vi "load_parameters.vi"(4 "Create Data Folder (T)":bool=TRUE, 5 "Set Up Projector and Camera (T)":bool=TRUE, 6 "additional loaded parameters to write":string[][](array[string]), 8 "error in (no error)":errorcluster, 9 "StimulusObject Parameters":variant, 10 "StimulusObjectClassInput":refnum<class "StimulusObject.lvclass">, 11 "Tags":string) -> (0 "error out":errorcluster, 2 "Computer Found":bool, 3 "Parameters":T1 {"FW_WormLengthSD" format="%#.6f"})   [LabVIEW 2019]
uses:
  Parameters.ctl
  StimulusObject.lvclass
  <vilib>/AdvancedString/Delimited String to 1D String Array.vi
  ParametersGlobal.vi
  <vilib>/Utility/file.llb/Write Delimited Spreadsheet (string).vi
  <vilib>/vision/driver/NI_Vision_Acquisition_Software.lvlib
  <vilib>/vision/NI_Vision_Development_Module.lvlib
panel:
  out "Cores Utilized":u32
  out "Camera Frame Rate":dbl
  # "Faux Worm Drawing"
  # "Tracking"
  # "Temporal Calibration"
  # "Stimulus Generation"
  # "Median Filtering"
  # "Experimental Settings"
  # "Camera and Projector Settings"
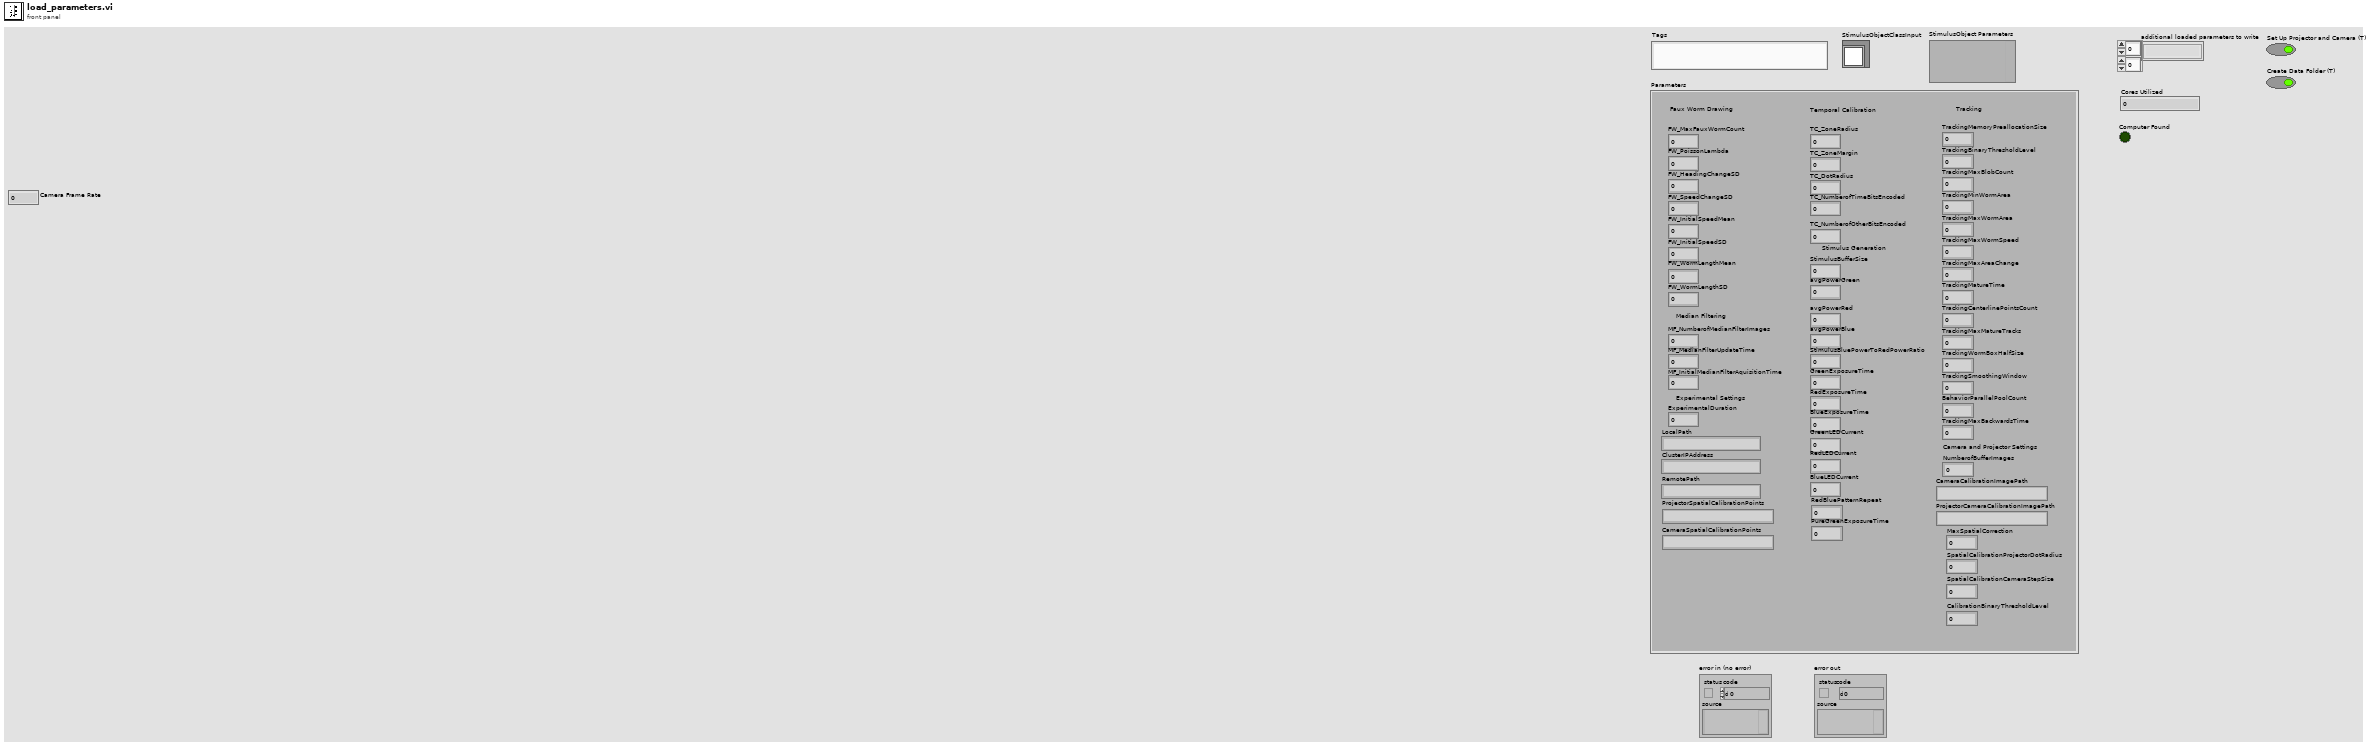
[diagram p1: front panel]
types:
  T1 = typedef "Parameters.ctl" = cluster{"FW_MaxFauxWormCount":i32, "FW_PoissonLambda":dbl, "FW_HeadingChangeSD":dbl, "FW_SpeedChangeSD":dbl, "FW_InitialSpeedMean":dbl, "FW_InitialSpeedSD":dbl, "FW_WormLengthMean":dbl, "FW_WormLengthSD":dbl, "MF_NumberofMedianFilterImages":i32, "MF_MedianFilterUpdateTime":i32, "MF_InitialMedianFilterAquisitionTime":dbl, "ExperimentalDuration":i32, "TC_ZoneRadius":i32, "TC_ZoneMargin":i32, "TC_DotRadius":dbl, "TC_NumberofTimeBitsEncoded":i32, "TC_NumberofOtherBitsEncoded":i32, "NumberofBufferImages":sgl, "CameraCalibrationImagePath":string, "ProjectorCameraCalibrationImagePath":string, "StimulusBufferSize":i32, "TrackingMemoryPreallocationSize":i32, "TrackingBinaryThresholdLevel":sgl, "TrackingMaxBlobCount":i32, "TrackingMinWormArea":dbl, "TrackingMaxWormArea":dbl, "TrackingMaxWormSpeed":dbl, "TrackingMaxAreaChange":dbl, "TrackingMatureTime":i32, "TrackingCenterlinePointsCount":i32, "TrackingMaxMatureTracks":i32, "TrackingWormBoxHalfSize":i32, "TrackingSmoothingWindow":i32, "BehaviorParallelPoolCount":i32, "LocalPath":string, "GreenExposureTime":i32, "RedExposureTime":i32, "BlueExposureTime":i32, "ClusterIPAddress":string, "RemotePath":string, "GreenLEDCurrent":u8, "RedLEDCurrent":u8, "BlueLEDCurrent":u8, "avgPowerGreen":sgl, "avgPowerRed":sgl, "avgPowerBlue":sgl, "StimulusBluePowerToRedPowerRatio":sgl, "TrackingMaxBackwardsTime":i32, "MaxSpatialCorrection":dbl, "ProjectorSpatialCalibrationPoints":string, "SpatialCalibrationProjectorDotRadius":i32, "SpatialCalibrationCameraStepSize":dbl, "CameraSpatialCalibrationPoints":string, "CalibrationBinaryThresholdLevel":dbl, "RedBluePatternRepeat":i32, "PureGreenExposureTime":i32}
  T2 = cluster{"Type":u32, "Version":u32, "Flags":u32, "SerialNumberHigh":u32, "SerialNumberLow":u32, "BusType":u32, "InterfaceName":string, "VendorName":string, "ModelName":string, "CameraFileName":string, "CameraAttributeURL":string}[]
  T3 = cluster{"Type":u32, "Version":u32, "Flags":u32, "SerialNumberHigh":u32, "SerialNumberLow":u32, "BusType":u32, "InterfaceName":string, "VendorName":string, "ModelName":string, "CameraFileName":string, "CameraAttributeURL":string}
  T4 = typedef "IMAQ Image.ctl" = refnum<image>
  T5 = typedef "Image Type" = u32
  T6 = enum16{"open", "replace", "create", "open or create", "replace or create", "replace or create with confirmation"}
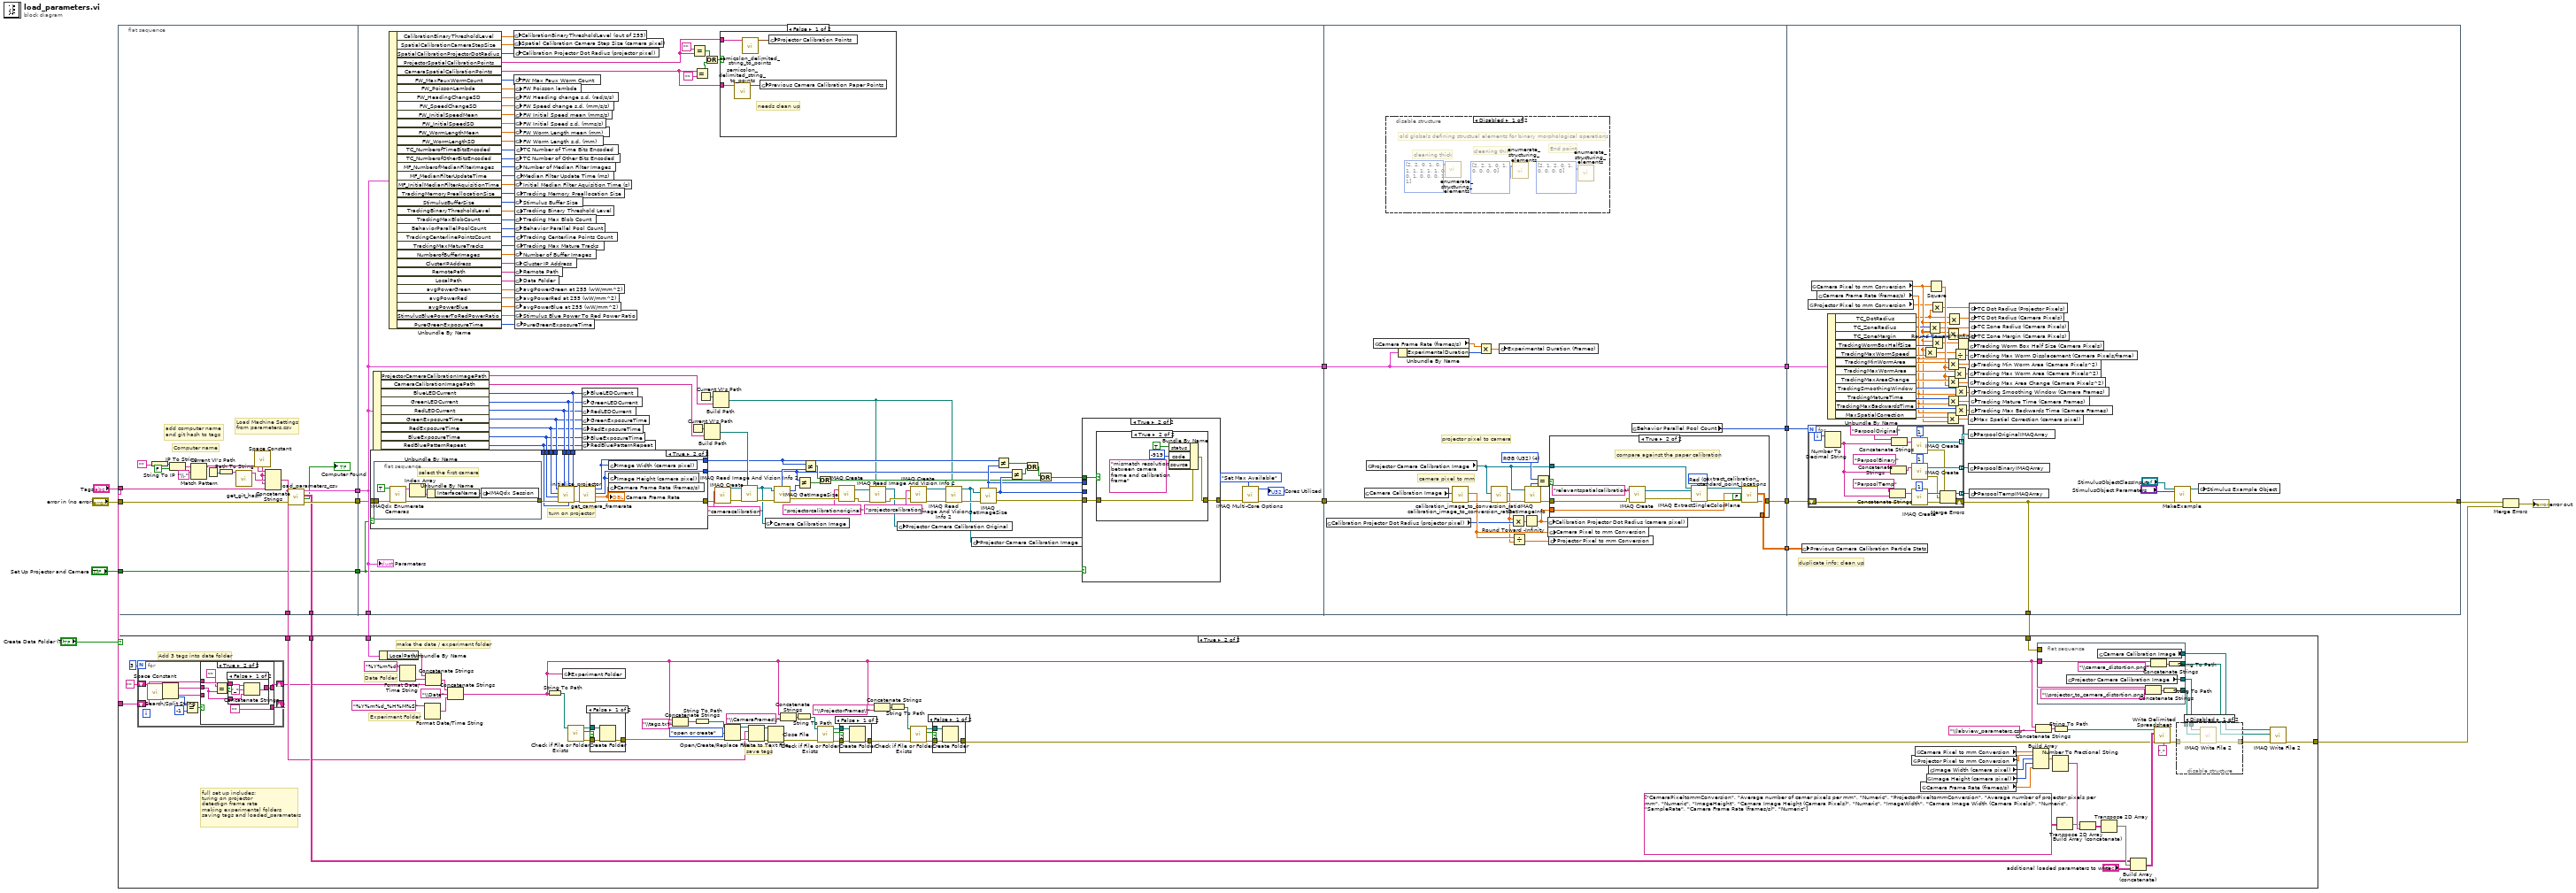
[diagram p0: block diagram]
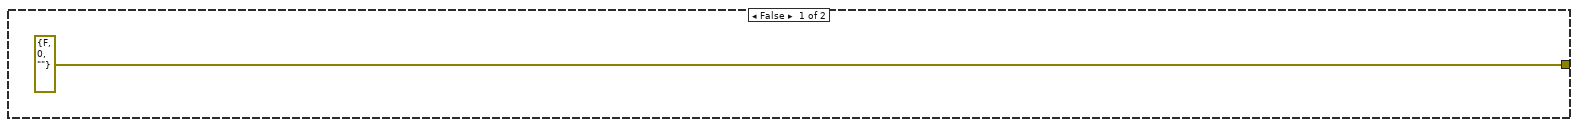
[diagram p2: hidden frame]
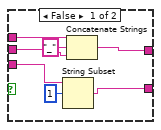
[diagram p7: hidden frame]
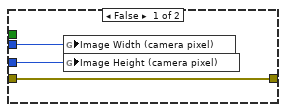
[diagram p10: hidden frame]
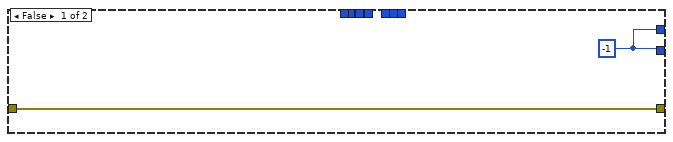
[diagram p12: hidden frame]
diagram:
  n1 = flat-sequence {
    tunnel: [w38] -> w19
    tunnel: "error in (no error)" -> [w23]
    tunnel: [w24] -> w18
    tunnel: "Tags" -> [w30]
    tunnel: [w26] -> w11
    tunnel: [w25] -> w10
    tunnel: [w22] -> w5
    tunnel: "Set Up Projector and Camera (T)" -> [w22]
    tunnel: w19 -> [w96]
    tunnel: [w87] -> w17
    tunnel: w18 -> [w97]
    tunnel: [w97] -> w14
    tunnel: [w97] -> w6
    tunnel: w5 -> [w73]
    tunnel: w17 -> [w187]
    tunnel: [w175] -> w16
    tunnel: [w183] -> w15
    tunnel: w14 -> [w183]
    tunnel: [w184] -> w13
    tunnel: [w172] -> w1
    tunnel: w16 -> [w226]
    tunnel: w15 -> [w247]
    tunnel: w13 -> [w225]
    tunnel: [w214] -> w9
    tunnel: [w218] -> w2
    tunnel: w1 -> [w217]
    frame #0 {
      # "add computer name \nand git hash to tags"
      # "Computer name"
      # "Load Machine Settings\nfrom parameters.csv"
      n2 = String To IP(1:"") -> (0:w37:u32)
      n3 = IP To String(1:FALSE, 2:w37) -> (0:w34:string)
      n4 = Match Pattern(string=w34, regular expression="\\.") -> (before substring=w28:string)  [unwired: 1 in, 3 out]
      n5 = Current VI's Path() -> (path=w32:path)
      n6 = Path To String(path=w32) -> (string=w31:string)
      n7 = call "get_git_hash.vi"("VI folder"=w31) -> ("github hash"=w29:string)  [unwired: 10 in]
      n8 = call <vilib>:"Space Constant.vi"() -> ("String"=w27:string)
      n9 = Concatenate Strings(w28, w27, w29, w27, w30) -> (w25:string)
      n10 = call "load_parameters_csv.vi"("error in (no error)"=w23, "Tags In"=w25) -> ("error out"=w38:errorcluster, "Computer Found"=→"Computer Found":bool, "Loaded Params"=w26:string[][], "Parameters Out"=w24:T1)  [unwired: 6 in]
    }
    frame #1 {
      n11 = Unbundle By Name(w97) -> ("ProjectorCameraCalibrationImagePath"=w67:string, "CameraCalibrationImagePath"=w119:string, "BlueLEDCurrent"=w46:u8, "GreenLEDCurrent"=w45:u8, "RedLEDCurrent"=w44:u8, "GreenExposureTime"=w43:i32, "RedExposureTime"=w42:i32, "BlueExposureTime"=w41:i32, "RedBluePatternRepeat"=w40:i32)
      n12 = case shown="True" w73 {
        tunnel: w96 -> [w146 w151]
        tunnel: [w146 w158] -> w95
        tunnel: w43 -> [_ w157]
        tunnel: w42 -> [_ w156]
        tunnel: w41 -> [_ w155]
        tunnel: w44 -> [_ w154]
        tunnel: w46 -> [_ w153]
        tunnel: w45 -> [_ w152]
        tunnel: [w145 w149] -> w66
        tunnel: [w145 w148] -> w65
        tunnel: w40 -> [_ w147]
        frame False {
          w145 = -1 ("Image Width (camera pixel)")
        }
        frame True {
          # "turn on projector"
          n13 = flat-sequence {
            tunnel: w151 -> [w163]
            tunnel: [w162] -> w150
            frame #0 {
              # "select the first camera"
              n14 = call <vilib>:"IMAQdx Enumerate Cameras.vi"("error in"=w163, "Connected Only? (Yes)"=TRUE) -> ("error out"=w162:errorcluster, "Camera Information Array"=w166:T2)  [unwired: 8 in]
              n15 = Index Array(array=w166) -> (element=w165:T3)  [unwired: 1 in]
              n16 = Unbundle By Name(w165) -> ("InterfaceName"=w161:string)
              n17 = global write "ParametersGlobal.vi" "IMAQdx Session"(w161) -> ()
            }
          }
          n18 = call "initialize_projector.vi"("BlueCurrent"=w153, "RedBluePatternRepeat"=w147, "GreenCurrent"=w152, "RedCurrent"=w154, "error in"=w150, "blue exp_time_us"=w155, "red exp_time_us"=w156, "green exp_time_us"=w157) -> ("error out"=w159:errorcluster)  [unwired: 3 in]
          n19 = call "get_camera_framerate.vi"("error in"=w159) -> ("error out"=w158:errorcluster, "Camera Frame Rate"=w160:dbl, "Y Resolution"=w148:i32, "X Resolution"=w149:i32)  [unwired: 7 in]
          "Camera Frame Rate" <- w160
          n20 = global write "ParametersGlobal.vi" "Image Width (camera pixel)"(w149) -> ()
          n21 = global write "ParametersGlobal.vi" "Image Height (camera pixel)"(w148) -> ()
          n22 = global write "ParametersGlobal.vi" "Camera Frame Rate (frames/s)"(w160) -> ()
        }
      }
      n23 = Unbundle By Name(w97) -> ("CalibrationBinaryThresholdLevel"=w47:dbl, "SpatialCalibrationCameraStepSize"=w61:dbl, "SpatialCalibrationProjectorDotRadius"=w62:i32, "ProjectorSpatialCalibrationPoints"=w63:string, "CameraSpatialCalibrationPoints"=w48:string, "FW_MaxFauxWormCount"=w109:i32, "FW_PoissonLambda"=w110:dbl, "FW_HeadingChangeSD"=w111:dbl, "FW_SpeedChangeSD"=w112:dbl, "FW_InitialSpeedMean"=w113:dbl, "FW_InitialSpeedSD"=w114:dbl, "FW_WormLengthMean"=w115:dbl, "FW_WormLengthSD"=w116:dbl, "TC_NumberofTimeBitsEncoded"=w117:i32, "TC_NumberofOtherBitsEncoded"=w118:i32, "MF_NumberofMedianFilterImages"=w108:i32, "MF_MedianFilterUpdateTime"=w107:i32, "MF_InitialMedianFilterAquisitionTime"=w106:dbl, "TrackingMemoryPreallocationSize"=w105:i32, "StimulusBufferSize"=w104:i32, "TrackingBinaryThresholdLevel"=w103:sgl, "TrackingMaxBlobCount"=w102:i32, "BehaviorParallelPoolCount"=w101:i32, "TrackingCenterlinePointsCount"=w100:i32, "TrackingMaxMatureTracks"=w99:i32, "NumberofBufferImages"=w98:sgl, "ClusterIPAddress"=w94:string, "RemotePath"=w93:string, "LocalPath"=w92:string, "avgPowerGreen"=w88:sgl, "avgPowerRed"=w89:sgl, "avgPowerBlue"=w90:sgl, "StimulusBluePowerToRedPowerRatio"=w91:sgl, "PureGreenExposureTime"=w39:i32)
      n24 = global write "ParametersGlobal.vi" "CalibrationBinaryThresholdLevel (out of 255)"(w47) -> ()
      n25 = global write "ParametersGlobal.vi" "Spatial Calibration Camera Step Size (camera pixel)"(w61) -> ()
      n26 = global write "ParametersGlobal.vi" "Calibration Projector Dot Radius (projector pixel)"(w62) -> ()
      n27 = global write "ParametersGlobal.vi" "FW Max Faux Worm Count"(w109) -> ()
      n28 = global write "ParametersGlobal.vi" "FW Poisson lambda"(w110) -> ()
      n29 = global write "ParametersGlobal.vi" "FW Heading change s.d. (rad/s/s)"(w111) -> ()
      n30 = global write "ParametersGlobal.vi" "FW Speed change s.d. (mm/s/s)"(w112) -> ()
      n31 = global write "ParametersGlobal.vi" "FW Initial Speed mean (mms/s)"(w113) -> ()
      n32 = global write "ParametersGlobal.vi" "FW Initial Speed s.d. (mms/s)"(w114) -> ()
      n33 = global write "ParametersGlobal.vi" "FW Worm Length mean (mm)"(w115) -> ()
      n34 = global write "ParametersGlobal.vi" "FW Worm Length s.d. (mm)"(w116) -> ()
      n35 = global write "ParametersGlobal.vi" "TC Number of Other Bits Encoded"(w118) -> ()
      n36 = global write "ParametersGlobal.vi" "Number of Median Filter Images"(w108) -> ()
      n37 = global write "ParametersGlobal.vi" "Initial Median Filter Aquisition Time (s)"(w106) -> ()
      n38 = global write "ParametersGlobal.vi" "Stimulus Buffer Size"(w104) -> ()
      n39 = global write "ParametersGlobal.vi" "Tracking Max Blob Count"(w102) -> ()
      n40 = global write "ParametersGlobal.vi" "Behavior Parallel Pool Count"(w101) -> ()
      n41 = global write "ParametersGlobal.vi" "Number of Buffer Images"(w98) -> ()
      n42 = global write "ParametersGlobal.vi" "Cluster IP Address"(w94) -> ()
      n43 = global write "ParametersGlobal.vi" "Remote Path"(w93) -> ()
      n44 = global write "ParametersGlobal.vi" "Data Folder"(w92) -> ()
      n45 = global write "ParametersGlobal.vi" "avgPowerGreen at 255 (wW/mm^2)"(w88) -> ()
      n46 = global write "ParametersGlobal.vi" "avgPowerRed at 255 (wW/mm^2)"(w89) -> ()
      n47 = global write "ParametersGlobal.vi" "avgPowerBlue at 255 (wW/mm^2)"(w90) -> ()
      n48 = global write "ParametersGlobal.vi" "Stimulus Blue Power To Red Power Ratio"(w91) -> ()
      n49 = global write "ParametersGlobal.vi" "TC Number of Time Bits Encoded"(w117) -> ()
      n50 = global write "ParametersGlobal.vi" "Median Filter Update Time (ms)"(w107) -> ()
      n51 = global write "ParametersGlobal.vi" "Tracking Memory Preallocation Size"(w105) -> ()
      n52 = global write "ParametersGlobal.vi" "Tracking Binary Threshold Level"(w103) -> ()
      n53 = global write "ParametersGlobal.vi" "Tracking Centerline Points Count"(w100) -> ()
      n54 = global write "ParametersGlobal.vi" "Tracking Max Mature Tracks"(w99) -> ()
      n55 = global write "ParametersGlobal.vi" "PureGreenExposureTime"(w39) -> ()
      n56 = global write "ParametersGlobal.vi" "BlueLEDCurrent"(w46) -> ()
      n57 = global write "ParametersGlobal.vi" "GreenLEDCurrent"(w45) -> ()
      n58 = global write "ParametersGlobal.vi" "RedLEDCurrent"(w44) -> ()
      n59 = global write "ParametersGlobal.vi" "GreenExposureTime"(w43) -> ()
      n60 = global write "ParametersGlobal.vi" "RedExposureTime"(w42) -> ()
      n61 = global write "ParametersGlobal.vi" "BlueExposureTime"(w41) -> ()
      n62 = global write "ParametersGlobal.vi" "RedBluePatternRepeat"(w40) -> ()
      n63 = Current VI's Path() -> (path=w124:path)
      n64 = Equal?(x="", y=w63) -> (x = y?=w51:bool)
      n65 = Equal?(x=w48, y="") -> (x = y?=w50:bool)
      n66 = Current VI's Path() -> (path=w128:path)
      n67 = Or(x=w51, y=w50) -> (x .or. y?=w49:bool)
      n68 = Build Path(base path=w124, name or relative path=w119) -> (appended path=w121:path)
      n69 = Build Path(base path=w128, name or relative path=w67) -> (appended path=w54:path)
      n70 = call "IMAQ Create"("Image Name"="cameracalibration", "error in (no error)"=w95) -> ("New Image"=w123:T4, "error out"=w122:errorcluster)  [unwired: 3 in]
      n71 = case shown="False" w49 {
        tunnel: w63 -> [w132 _]
        tunnel: w48 -> [w130 _]
        frame False {
          # "needs clean up"
          n72 = call "semicolon_delimited_string_to_points.vi"("delimited string"=w130) -> ("Array"=w129:cluster{"X":dbl, "Y":dbl}[])  [unwired: 10 in]
          n73 = call "semicolon_delimited_string_to_points.vi"("delimited string"=w132) -> ("Array"=w131:cluster{"X":dbl, "Y":dbl}[])  [unwired: 10 in]
          n74 = global write "ParametersGlobal.vi" "Previous Camera Calibration Paper Points"(w129) -> ()
          n75 = global write "ParametersGlobal.vi" "Projector Calibration Points"(w131) -> ()
        }
        frame True {
        }
      }
      n76 = call "IMAQ Read Image And Vision Info 2"("File Path"=w121, "error in (no error)"=w122, "Image"=w123) -> ("error out"=w84:errorcluster, "Image Out"=w81:T4)  [unwired: 6 in, 1 out]
      n77 = global write "ParametersGlobal.vi" "Camera Calibration Image"(w81) -> ()
      n78 = call "IMAQ GetImageSize"("Image"=w81, "error in (no error)"=w84) -> ("Y Resolution"=w82:i32, "X Resolution"=w83:i32, "error out"=w59:errorcluster)  [unwired: 2 in]
      n79 = Not Equal?(x=w65, y=w82) -> (x != y?=w78:bool)
      n80 = Not Equal?(x=w66, y=w83) -> (x != y?=w77:bool)
      n81 = Or(x=w77, y=w78) -> (x .or. y?=w60:bool)
      n82 = call "IMAQ Create"("Image Name"="projectorcalibrationoriginal", "error in (no error)"=w59) -> ("New Image"=w56:T4, "error out"=w57:errorcluster)  [unwired: 3 in]
      n83 = call "IMAQ Read Image And Vision Info 2"("File Path"=w54, "error in (no error)"=w57, "Image"=w56) -> ("error out"=w55:errorcluster, "Image Out"=w53:T4)  [unwired: 6 in, 1 out]
      n84 = global write "ParametersGlobal.vi" "Projector Camera Calibration Original"(w53) -> ()
      n85 = call "IMAQ Create"("Image Name"="projectorcalibration", "error in (no error)"=w55) -> ("New Image"=w126:T4, "error out"=w125:errorcluster)  [unwired: 3 in]
      n86 = call "IMAQ Read Image And Vision Info 2"("File Path"=w54, "error in (no error)"=w125, "Image"=w126) -> ("error out"=w80:errorcluster, "Image Out"=w79:T4)  [unwired: 6 in, 1 out]
      n87 = global write "ParametersGlobal.vi" "Projector Camera Calibration Image"(w79) -> ()
      n88 = call "IMAQ GetImageSize"("Image"=w79, "error in (no error)"=w80) -> ("Y Resolution"=w70:i32, "X Resolution"=w69:i32, "error out"=w72:errorcluster)  [unwired: 2 in]
      n89 = Not Equal?(x=w66, y=w69) -> (x != y?=w76:bool)
      n90 = Not Equal?(x=w65, y=w70) -> (x != y?=w75:bool)
      n91 = Or(x=w76, y=w75) -> (x .or. y?=w74:bool)
      n92 = Or(x=w74, y=w60) -> (x .or. y?=w68:bool)
      n93 = case shown="True" w73 {
        tunnel: w72 -> [w135 w137]
        tunnel: [w135 w136] -> w71
        tunnel: w70 -> [w134 _]
        tunnel: w69 -> [w133 _]
        tunnel: w68 -> [_ w138]
        frame False {
          n94 = global write "ParametersGlobal.vi" "Image Width (camera pixel)"(w133) -> ()
          n95 = global write "ParametersGlobal.vi" "Image Height (camera pixel)"(w134) -> ()
        }
        frame True {
          n96 = case shown="True" w138 {
            tunnel: w137 -> [w139 w141]
            tunnel: [w139 w140] -> w136
            frame False {
              # "all resolutions match"
            }
            frame True {
              n97 = Bundle By Name(cluster=w141, "status"=TRUE, "code"=-919, "source"="mismatch resolution between camera frame and calibration frame") -> (w140:errorcluster)
            }
          }
        }
      }
      n98 = call "IMAQ Multi-Core Options"("Get/Set Number of Cores (Get)"=enum32{"Get", "Set", "Set Max Available"}."Set Max Available", "error in (no error)"=w71) -> ("error out"=w87:errorcluster, "Cores Utilized"=→"Cores Utilized":u32)  [unwired: 8 in]
      "Parameters" <- w97
    }
    frame #2 {
      w176 = T5 4 items=["Grayscale (U8)", "Grayscale (I16)", "Grayscale (SGL)", "Complex (CSG)", "RGB (U32)", "HSL (U32)", "RGB (U64)", "Grayscale (U16)"] ("Image Type")
      # "projector pixel to camera"
      # "camera pixel to mm"
      n99 = global read "ParametersGlobal.vi" "Calibration Projector Dot Radius (projector pixel)"() -> (w170:i32)
      n100 = global read "ParametersGlobal.vi" "Camera Calibration Image"() -> (w186:T4)
      n101 = global read "ParametersGlobal.vi" "Projector Camera Calibration Image"() -> (w171:T4)
      n102 = global read "ParametersGlobal.vi" "Camera Frame Rate (frames/s)"() -> (w182:sgl)
      n103 = disable-structure shown="Disabled" {
        frame Disabled {
          # "old globals defining structual elements for binary morphological operations"
          # "End point"
          # "cleaning thin"
          # "cleaning thick"
          n104 = call "enumerate_structuring_elements.vi"("Structuring Elements"=i32[][][] [[[2, 2, 0], [1, 0, 1], [1, 1, 1]], [[1, 0, 0], [1, 0, 0], [0, 1, 1]]]) -> ()  [unwired: 4 in, 1 out]
          n105 = call "enumerate_structuring_elements.vi"("Structuring Elements"=i32[][][] [[[2, 2, 1], [0, 1, 0], [0, 0, 0]]]) -> ()  [unwired: 4 in, 1 out]
          n106 = call "enumerate_structuring_elements.vi"("Structuring Elements"=i32[][][] [[[2, 1, 2], [0, 1, 0], [0, 0, 0]]]) -> ()  [unwired: 4 in, 1 out]
        }
        frame Enabled {
        }
      }
      n107 = Unbundle By Name(w183) -> ("ExperimentalDuration"=w181:i32)
      n108 = call "calibration_image_to_conversion_ratio.vi"("error in (no error)"=w187, "Calibration Image"=w186) -> ("error out"=w188:errorcluster, "conversion ratio"=w179:dbl)  [unwired: 8 in]
      n109 = Multiply(x=w182, y=w181) -> (x*y=w180:sgl)
      n110 = call "calibration_image_to_conversion_ratio.vi"("error in (no error)"=w188, "Calibration Image"=w171) -> ("error out"=w178:errorcluster, "conversion ratio"=w169:dbl)  [unwired: 8 in]
      n111 = global write "ParametersGlobal.vi" "Experimental Duration (Frames)"(w180) -> ()
      n112 = Multiply(x=w169, y=w170) -> (x*y=w168:dbl)
      n113 = Divide(x=w179, y=w169) -> (x/y=w185:dbl)
      n114 = Round Toward -Infinity(1:w168) -> (0:w167:dbl)
      n115 = call "IMAQ GetImageInfo"("error in (no error)"=w178, "Image"=w171) -> ("error out"=w174:errorcluster, "Image Type"=w177:T5)  [unwired: 2 in, 6 out]
      n116 = Equal?(x=w176, y=w177) -> (x = y?=w173:bool)
      n117 = global write "ParametersGlobal.vi" "Calibration Projector Dot Radius (camera pixel)"(w167) -> ()
      n118 = global write "ParametersGlobal.vi" "Camera Pixel to mm Conversion"(w179) -> ()
      n119 = global write "ParametersGlobal.vi" "Projector Pixel to mm Conversion"(w185) -> ()
      n120 = case shown="True" w173 {
        tunnel: [w189 w195] -> w175
        tunnel: w174 -> [w189 w199]
        tunnel: w171 -> [_ w196]
        tunnel: [_ w197] -> w172
        tunnel: w167 -> [_ w194]
        frame False {
        }
        frame True {
          w191 = 0 items=["Red", "Green", "Blue", "Hue", "Saturation", "Luminance", "Value", "Intensity"] ("Color Plane")
          # "compare against the paper calibration"
          n121 = call "IMAQ Create"("Image Name"="relevantspatialcalibration", "error in (no error)"=w199) -> ("New Image"=w192:T4, "error out"=w193:errorcluster)  [unwired: 3 in]
          n122 = call "IMAQ ExtractSingleColorPlane"("Color Plane"=w191, "error in (no error)"=w193, "Image Dst"=w192, "Image Src"=w196) -> ("error out"=w200:errorcluster, "Image Dst Out"=w201:T4)  [unwired: 6 in]
          n123 = call "extract_calibration_standard_point_locations.vi"("error in (no error)"=w200, "Agar (T) Paper (F)"=FALSE, "expected dot radius (camera pixels)"=w194, "Image Src"=w201) -> ("error out"=w195:errorcluster, "Particle Measurements (Pixels)"=w197:dbl[][])  [unwired: 5 in, 1 out]
        }
      }
      n124 = global read "ParametersGlobal.vi" "Behavior Parallel Pool Count"() -> (w184:i32)
    }
    frame #3 {
      # "duplicate info: clean up"
      n125 = global write "ParametersGlobal.vi" "Previous Camera Calibration Particle Stats"(w217) -> ()
      n126 = global read "ParametersGlobal.vi" "Projector Pixel to mm Conversion"() -> (w206:sgl)
      n127 = for {
        N: w225 -> [_]
        shift-right: [w260] -> w218
        shift-left: w226 -> [w251]
        tunnel: [w264] -> w227 mode=indexing
        tunnel: [w259] -> w228 mode=indexing
        tunnel: [w256] -> w229 mode=indexing
        i -> [w261]
        n128 = Number To Decimal String(number=w261) -> (decimal integer string=w255:string)  [unwired: 1 in]
        n129 = Concatenate Strings("ParpoolTemp", w255) -> (w258:string)
        n130 = Concatenate Strings("ParpoolBinary", w255) -> (w262:string)
        n131 = Concatenate Strings("ParpoolOriginal", w255) -> (w265:string)
        n132 = call "IMAQ Create"("Border Size"=1, "Image Name"=w262) -> ("New Image"=w259:T4, "error out"=w253:errorcluster)  [unwired: 3 in]
        n133 = call "IMAQ Create"("Border Size"=1, "Image Name"=w258, "error in (no error)"=w251) -> ("New Image"=w256:T4, "error out"=w254:errorcluster)  [unwired: 2 in]
        n134 = call "IMAQ Create"("Border Size"=1, "Image Name"=w265) -> ("New Image"=w264:T4, "error out"=w252:errorcluster)  [unwired: 3 in]
        n135 = Merge Errors(w252, w253, w254) -> (w260:errorcluster)
      }
      n136 = global read "ParametersGlobal.vi" "Camera Pixel to mm Conversion"() -> (w211:sgl)
      n137 = global read "ParametersGlobal.vi" "Camera Frame Rate (frames/s)"() -> (w221:sgl)
      n138 = Unbundle By Name(w247) -> ("TC_DotRadius"=w207:dbl, "TC_ZoneRadius"=w213:i32, "TC_ZoneMargin"=w212:i32, "TrackingWormBoxHalfSize"=w236:i32, "TrackingMaxWormSpeed"=w239:dbl, "TrackingMinWormArea"=w246:dbl, "TrackingMaxWormArea"=w245:dbl, "TrackingMaxAreaChange"=w242:dbl, "TrackingSmoothingWindow"=w233:i32, "TrackingMatureTime"=w231:i32, "TrackingMaxBackwardsTime"=w222:i32, "MaxSpatialCorrection"=w216:dbl)
      n139 = Multiply(x=w211, y=w239) -> (x*y=w238:dbl)
      n140 = Multiply(x=w213, y=w211) -> (x*y=w209:sgl)
      n141 = Square(x=w211) -> (x^2=w241:sgl)
      n142 = Multiply(x=w206, y=w207) -> (x*y=w205:dbl)
      n143 = Multiply(x=w211, y=w236) -> (x*y=w235:sgl)
      n144 = Multiply(x=w216, y=w211) -> (x*y=w215:dbl)
      n145 = Multiply(x=w211, y=w212) -> (x*y=w208:sgl)
      n146 = Multiply(x=w246, y=w241) -> (x*y=w244:dbl)
      n147 = Multiply(x=w242, y=w241) -> (x*y=w240:dbl)
      n148 = Multiply(x=w231, y=w221) -> (x*y=w230:sgl)
      n149 = Multiply(x=w207, y=w211) -> (x*y=w210:dbl)
      n150 = Multiply(x=w245, y=w241) -> (x*y=w243:dbl)
      n151 = Divide(x=w238, y=w221) -> (x/y=w237:dbl)
      n152 = Multiply(x=w233, y=w221) -> (x*y=w232:sgl)
      n153 = Multiply(x=w222, y=w221) -> (x*y=w220:sgl)
      n154 = Round Toward +Infinity(x=w235) -> (ceil(x): smallest int >= x=w234:sgl)
      n155 = global write "ParametersGlobal.vi" "Tracking Worm Box Half Size (Camera Pixels)"(w234) -> ()
      n156 = global write "ParametersGlobal.vi" "Tracking Max Worm Displacement (Camera Pixels/frame)"(w237) -> ()
      n157 = global write "ParametersGlobal.vi" "Tracking Max Worm Area (Camera Pixels^2)"(w243) -> ()
      n158 = global write "ParametersGlobal.vi" "Tracking Max Area Change (Camera Pixels^2)"(w240) -> ()
      n159 = global write "ParametersGlobal.vi" "Max Spatial Correction (camera pixel)"(w215) -> ()
      n160 = global write "ParametersGlobal.vi" "ParpoolOriginalIMAQArray"(w227) -> ()
      n161 = global write "ParametersGlobal.vi" "ParpoolBinaryIMAQArray"(w228) -> ()
      n162 = global write "ParametersGlobal.vi" "TC Dot Radius (Projector Pixels)"(w205) -> ()
      n163 = global write "ParametersGlobal.vi" "TC Dot Radius (Camera Pixels)"(w210) -> ()
      n164 = global write "ParametersGlobal.vi" "TC Zone Radius (Camera Pixels)"(w209) -> ()
      n165 = global write "ParametersGlobal.vi" "TC Zone Margin (Camera Pixels)"(w208) -> ()
      n166 = global write "ParametersGlobal.vi" "Tracking Min Worm Area (Camera Pixels^2)"(w244) -> ()
      n167 = global write "ParametersGlobal.vi" "Tracking Smoothing Window (Camera Frames)"(w232) -> ()
      n168 = global write "ParametersGlobal.vi" "ParpoolTempIMAQArray"(w229) -> ()
      n169 = global write "ParametersGlobal.vi" "Tracking Mature Time (Camera Frames)"(w230) -> ()
      n170 = global write "ParametersGlobal.vi" "Tracking Max Backwards Time (Camera Frames)"(w220) -> ()
      n171 = call-dynamic "MakeExample.vi"("error in (no error)"=w218, "StimulusObject Parameters"="StimulusObject Parameters", "StimulusObject in"="StimulusObjectClassInput") -> ("error out"=w214:errorcluster, "StimulusObject out"=w223:refnum<class "StimulusObject.lvclass">)  [unwired: 7 in]
      n172 = global write "ParametersGlobal.vi" "Stimulus Example Object"(w223) -> ()
    }
  }
  n173 = case shown="True" "Create Data Folder (T)" {
    tunnel: "Tags" -> [_ w335]
    tunnel: w11 -> [_ w284]
    tunnel: w10 -> [_ w282]
    tunnel: [errorcluster {"status"=FALSE, "code"=0, "source"=""} ("error out") w275] -> w7
    tunnel: w6 -> [_ w279]
    tunnel: w2 -> [_ w268]
    frame False {
    }
    frame True {
      # "full set up includes:\nturing on projector\ndetectign frame rate\nmaking experimental folders\nsaving tags and loaded_parameters"
      # "save tags"
      # "make the date / experiment folder"
      # "Experiment Folder"
      # "Date Folder"
      # "Add 3 tags into date folder"
      n174 = for {
        N: 3 -> [_]
        shift-right: [w362] -> _
        shift-left: w335 -> [w371]
        shift-right: [w364] -> w278
        shift-left: "" -> [w369]
        n175 = call <vilib>:"Space Constant.vi"() -> ("String"=w370:string)
        n176 = Search/Split String(string=w371, search string/char (-)=w370) -> (substring before match=w368:string, match + rest of string=w367:string, offset of match=w366:i32)  [unwired: 1 in]
        n177 = Equal?(x=w366, y=-1) -> (x = y?=w363:bool)
        n178 = case shown="True" w363 {
          tunnel: w369 -> [w372 w382]
          tunnel: w368 -> [w373 w379]
          tunnel: w367 -> [w374 _]
          tunnel: [w376 ""] -> w362
          tunnel: [w375 w381] -> w364
          frame False {
            n179 = String Subset(string=w374, offset (0)=1) -> (substring=w376:string)  [unwired: 1 in]
            n180 = Concatenate Strings(w372, "_", w373) -> (w375:string)
          }
          frame True {
            n181 = Equal?(x="", y=w379) -> (x = y?=w383:bool)
            n182 = case shown="False" w383 {
              tunnel: w382 -> [w386 w389]
              tunnel: [w387 w389] -> w381
              tunnel: w379 -> [w385 _]
              frame False {
                n183 = Concatenate Strings(w386, "_", w385) -> (w387:string)
              }
              frame True {
              }
            }
          }
        }
      }
      n184 = Unbundle By Name(w279) -> ("LocalPath"=w269:string)
      n185 = Format Date/Time String(time format string (%c)="%Y%m%d") -> (date/time string=w330:string)  [unwired: 2 in]
      n186 = Format Date/Time String(time format string (%c)="%Y%m%d_%H%M%S") -> (date/time string=w329:string)  [unwired: 2 in]
      n187 = Concatenate Strings(w269, w330, w278) -> (w331:string)
      n188 = Concatenate Strings(w331, "\\Data", w329) -> (w270:string)
      n189 = String To Path(string=w270) -> (path=w328:path)
      n190 = global write "ParametersGlobal.vi" "Experiment Folder"(w270) -> ()
      n191 = call <vilib>:"Check if File or Folder Exists.vi"("path"=w328) -> ("error out"=w332:errorcluster, "file or folder exists?"=w326:bool, "dup path"=w327:path)  [unwired: 8 in]
      n192 = case shown="False" w326 {
        tunnel: w327 -> [w360 _]
        tunnel: [w359 w361] -> w308
        tunnel: w332 -> [w358 w361]
        frame False {
          n193 = Create Folder(path (use dialog)=w360, error in=w358) -> (error out=w359:errorcluster)  [unwired: 1 in, 2 out]
        }
        frame True {
        }
      }
      n194 = Concatenate Strings(w270, "\\tags.txt" ("string")) -> (w312:string)
      n195 = String To Path(string=w312) -> (path=w315:path)
      n196 = Open/Create/Replace File(file path (use dialog)=w315, error in=w308, operation (0:open)=T6."open or create") -> (refnum out=w314:refnum<file>, error out=w313:errorcluster)  [unwired: 3 in, 1 out]
      n197 = Write to Text File(file (use dialog)=w314, text=w282, error in=w313) -> (refnum out=w316:refnum<file>, error out=w317:errorcluster)  [unwired: 1 in, 1 out]
      n198 = Close File(refnum=w316, error in=w317) -> (error out=w320:errorcluster)  [unwired: 1 out]
      n199 = Concatenate Strings(w270, "\\CameraFrames\\" ("string")) -> (w321:string)
      n200 = String To Path(string=w321) -> (path=w322:path)
      n201 = call <vilib>:"Check if File or Folder Exists.vi"("error in (no error)"=w320, "path"=w322) -> ("error out"=w323:errorcluster, "file or folder exists?"=w319:bool, "dup path"=w318:path)  [unwired: 7 in]
      n202 = case shown="False" w319 {
        tunnel: w318 -> [w356 _]
        tunnel: [w355 w357] -> w283
        tunnel: w323 -> [w354 w357]
        frame False {
          n203 = Create Folder(path (use dialog)=w356, error in=w354) -> (error out=w355:errorcluster)  [unwired: 1 in, 2 out]
        }
        frame True {
        }
      }
      n204 = Concatenate Strings(w270, "\\ProjectorFrames\\" ("string")) -> (w304:string)
      n205 = String To Path(string=w304) -> (path=w305:path)
      n206 = call <vilib>:"Check if File or Folder Exists.vi"("error in (no error)"=w283, "path"=w305) -> ("error out"=w306:errorcluster, "file or folder exists?"=w303:bool, "dup path"=w302:path)  [unwired: 7 in]
      n207 = case shown="False" w303 {
        tunnel: w302 -> [w352 _]
        tunnel: [w351 w353] -> w281
        tunnel: w306 -> [w350 w353]
        frame False {
          n208 = Create Folder(path (use dialog)=w352, error in=w350) -> (error out=w351:errorcluster)  [unwired: 1 in, 2 out]
        }
        frame True {
        }
      }
      n209 = global read "ParametersGlobal.vi" "Projector Pixel to mm Conversion"() -> (w292:sgl)
      n210 = global read "ParametersGlobal.vi" "Camera Pixel to mm Conversion"() -> (w291:sgl)
      n211 = global read "ParametersGlobal.vi" "Camera Frame Rate (frames/s)"() -> (w307:sgl)
      n212 = global read "ParametersGlobal.vi" "Image Height (camera pixel)"() -> (w294:i32)
      n213 = global read "ParametersGlobal.vi" "Image Width (camera pixel)"() -> (w293:i32)
      n214 = Build Array(w291, w292, w293, w294, w307) -> (w295:sgl[])
      n215 = Concatenate Strings(w270, "\\labview_parameters.csv" ("string")) -> (w289:string)
      n216 = flat-sequence {
        tunnel: [w349] -> w274
        tunnel: [w348] -> w273
        tunnel: [w343] -> w272
        tunnel: [w342] -> w271
        tunnel: w270 -> [w341]
        tunnel: w268 -> [_]
        frame #0 {
          n217 = global read "ParametersGlobal.vi" "Projector Camera Calibration Image"() -> (w349:T4)
          n218 = global read "ParametersGlobal.vi" "Camera Calibration Image"() -> (w348:T4)
          n219 = Concatenate Strings(w341, "\\projector_to_camera_distortion.png" ("string")) -> (w345:string)
          n220 = Concatenate Strings(w341, "\\camera_distortion.png" ("string")) -> (w347:string)
          n221 = String To Path(string=w345) -> (path=w343:path)
          n222 = String To Path(string=w347) -> (path=w342:path)
        }
      }
      n223 = Number To Fractional String(number=w295) -> (F-format string=w297:string[])  [unwired: 3 in]
      n224 = String To Path(string=w289) -> (path=w290:path)
      n225 = Transpose 2D Array(2D array=string[][] [["CameraPixeltommConversion", "Average number of camer pixels per mm", "Numeric"], ["ProjectorPixeltommConversion", "Average number of projector pixels per mm", "Numeric"], ["ImageHeight", "Camera Image Height (Camera Pixels)", "Numeric"], ["ImageWidth", "Camera Image Width (Camera Pixels)", "Numeric"], ["SampleRate", "Camera Frame Rate (frames/s)", "Numeric"]]) -> (transposed array=w296:string[][])
      n226 = Build Array (concatenate)(w296, w297) -> (w298:string[][])
      n227 = Transpose 2D Array(2D array=w298) -> (transposed array=w299:string[][])
      n228 = Build Array (concatenate)(w284, w299, "additional loaded parameters to write") -> (w301:string[][])
      n229 = call-poly <vilib>:"Write Delimited Spreadsheet.vi"("file path (dialog if empty)"=w290, "2D data"=w301, "error in (no error)"=w281, "delimiter (\\t)"="," ("delimiter (\\t)")) -> ("error out"=w277:errorcluster)  [unwired: 10 in, 1 out]
      n230 = disable-structure shown="Disabled" {
        disable-tunnel: w277 -> [w339 w340]
        disable-tunnel: [w338 w340] -> w276
        disable-tunnel: w274 -> [w337 _]
        disable-tunnel: w272 -> [w336 _]
        frame Disabled {
          n231 = call-poly "IMAQ Write File 2"("error in (no error)"=w339, "File Path"=w336, "Image"=w337) -> ("error out"=w338:errorcluster)  [unwired: 7 in, 1 out]
        }
        frame Enabled {
        }
      }
      n232 = call-poly "IMAQ Write File 2"("error in (no error)"=w276, "File Path"=w271, "Image"=w273) -> ("error out"=w275:errorcluster)  [unwired: 7 in, 1 out]
    }
  }
  n233 = Merge Errors(w9, w7) -> (→"error out":errorcluster)
